vi "ElevFF_Calculate.vi"(9 "Accel":dbl, 10 "Velocity":dbl, 11 "in ELEV_FF":T1 {"Kg" format="%13.5p"; "Ka" format="%13.5p"; "Kv" format="%13.5p"; "Ks" format="%13.5p"}) -> (3 "FeedForward":dbl)   [LabVIEW 2019, in "Trajectory_Library.lvlib"]
doc: "Calculates the feedforward from the gains and setpoints.\n \nInputs: \n - ElevFF -- The ElevFF data cluster\n - velocity -- The velocity setpoint.\n - acceleration -- The acceleration setpoint.\n\nOutputs:\n - feedforward -- The computed feedforward."
uses:
  Trajectory_Library.lvlib
  TypeDef/ELEV_FF.ctl
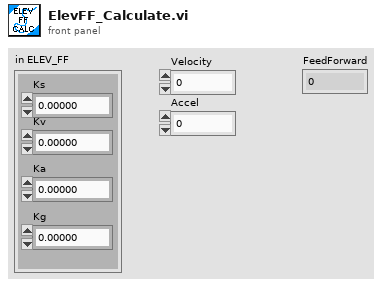
[diagram p1: front panel]
types:
  T1 = typedef "Trajectory_Library.lvlib/ELEV_FF.ctl" = cluster{"Ks":dbl, "Kv":dbl, "Ka":dbl, "Kg":dbl}
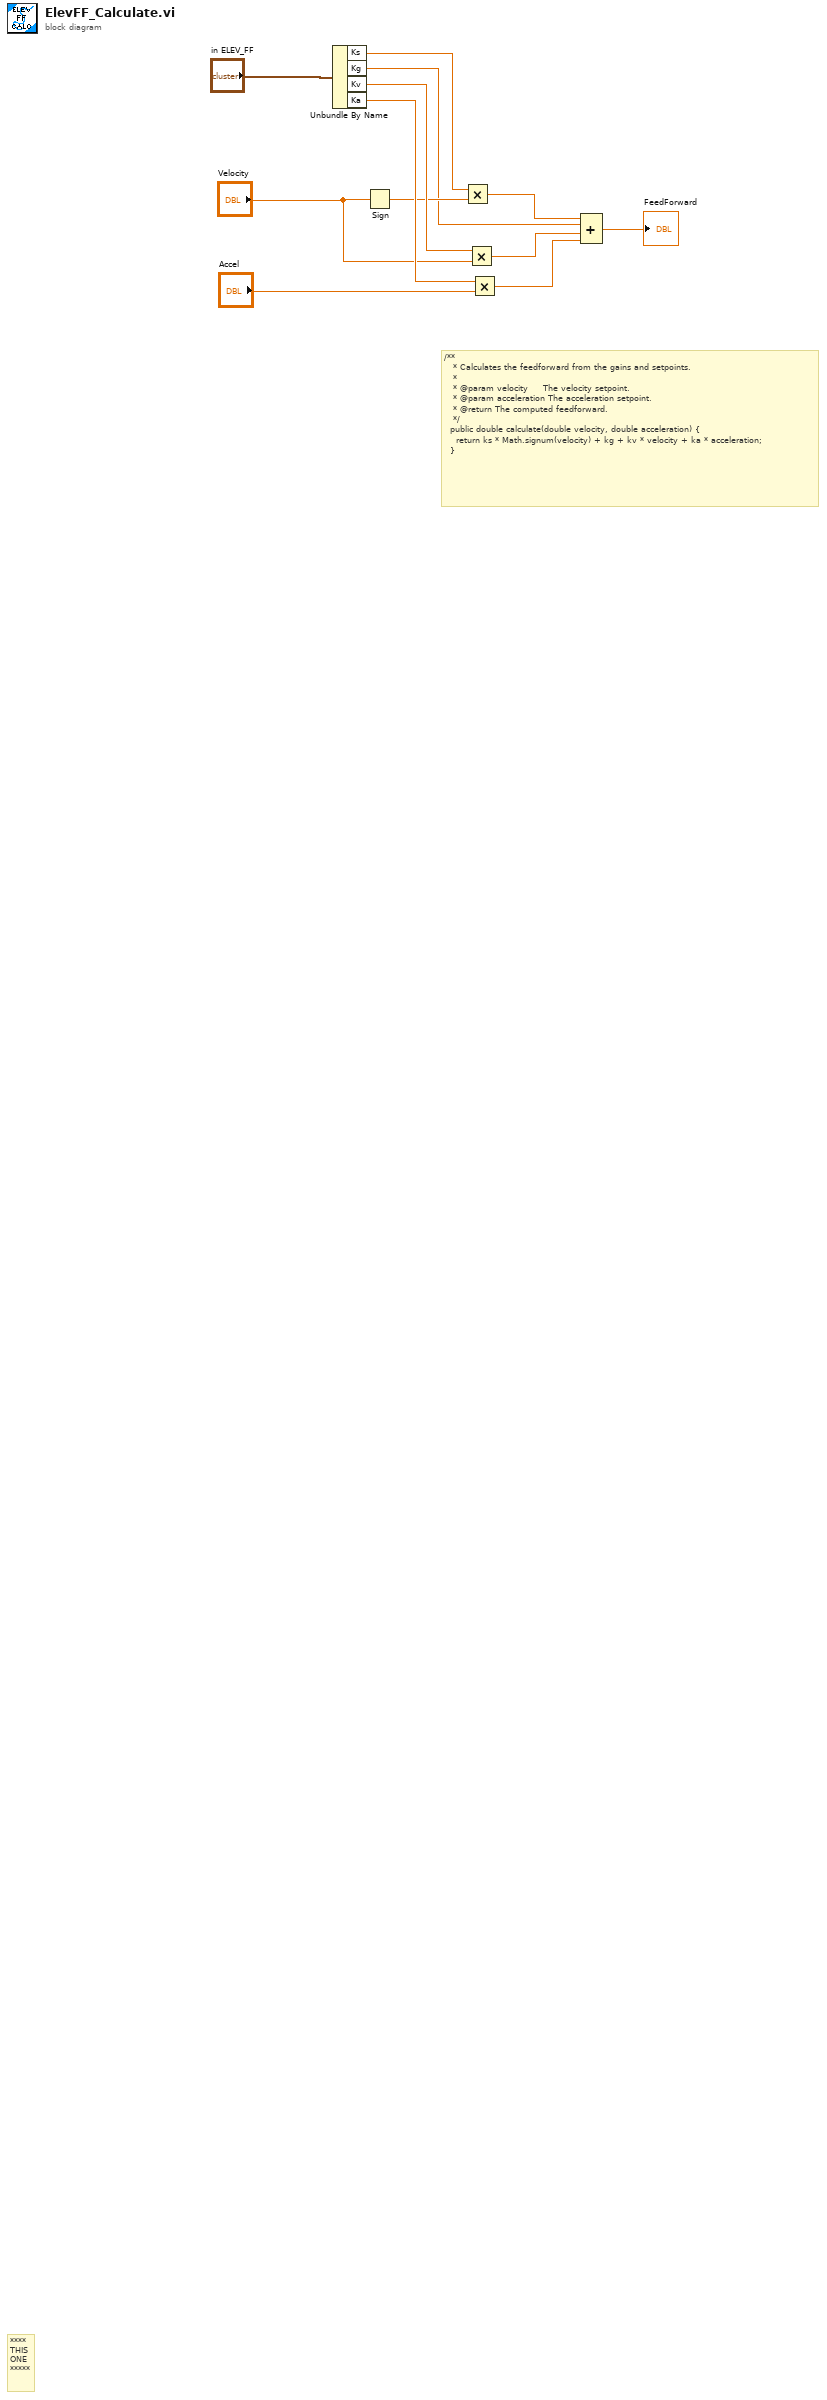
[diagram p0: block diagram]
diagram:
  # "/**\n   * Calculates the feedforward from the gains and setpoints.\n   *\n   * @param velocity     The velocity setpoint.\n   * @param acceleration The acceleration setpoint.\n   * @return The computed feedforward.\n   */\n  public double calculate(double velocity, double acceleration) {\n    return ks * Math.signum(velocity) + kg + kv * velocity + ka * acceleration;\n  }"
  # "****\nTHIS\nONE\n*****"
  n1 = Unbundle By Name("in ELEV_FF") -> ("Ks"=w7:dbl, "Kg"=w3:dbl, "Kv"=w6:dbl, "Ka"=w5:dbl)
  n2 = Sign(1:"Velocity") -> (0:w4:dbl)
  n3 = Multiply(x=w7, y=w4) -> (x*y=w10:dbl)
  n4 = Multiply(x=w6, y="Velocity") -> (x*y=w9:dbl)
  n5 = Multiply(x=w5, y="Accel") -> (x*y=w8:dbl)
  n6 = Compound Arithmetic op=ADD(w10, w3, w9, w8) -> (→"FeedForward":dbl)
